vi "Measurement Logic.vi"() -> ()   [LabVIEW 2021, in "adc_fullScaleError.lvlib"]
uses:
  adc_fullScaleError.lvlib
  <instrlib>/niDMM/nidmm.llb/niDMM Function.ctl
  <instrlib>/niDMM/nidmm.llb/niDMM Configure Measurement Digits.vi
  Controls/Sweep Transition Settings.ctl
  <vilib>/DAQmx/configure/timing.llb/DAQmx Timing (Sample Clock).vi
  <vilib>/DAQmx/create/channels.llb/DAQmx Create Channel (AO-Voltage-Basic).vi
  shared/digitalInterface/client/dcvmDPI_AD7606B_client/dcvmDPI_AD7606B_client.lvlib
  <vilib>/gRPC/LabVIEW gRPC Library/Shared/grpcId.ctl
  <vilib>/gRPC/LabVIEW gRPC Library/grpc-lvsupport-release.lvlib
  shared/digitalInterface/client/dcvmDPI_AD7606B_clientImpl/dcvmDPI_AD7606B_clientImpl.lvlib
  Measurement Configuration.ctl
  Measurement Results.ctl
  <vilib>/MeasurementLink/MeasurementLink Measurement Server/Measure Call Context/Measure Call Context.lvclass
panel:
  out "error out":errorcluster
  in  "error in":errorcluster
  out "measurement results":T1
  in  "measurement configuration":T2={"Input channel"=1, "Full scale range"=10.0, "Transition span"=1.5, "Transition step size"=0.05, "Analog source resource name"="", "Digital capture resource name"="", "Digital capture sample rate"=0.0, "Digital capture samples"=10000, "DMM resource name"="", "DMM range"=10.0, "DMM resolution"=5.5} {"DMM range" format="%#_6pV"; "Digital capture sample rate" format="%#_6pS/s"; "Transition step size" format="%#_gLSB"; "Transition span" format="%#_gLSB"; "Full scale range" format="%#_6pV"}
  out "measure call context out":refnum<class "Measure Call Context.lvclass">
  in  "measure call context in":refnum<class "Measure Call Context.lvclass">
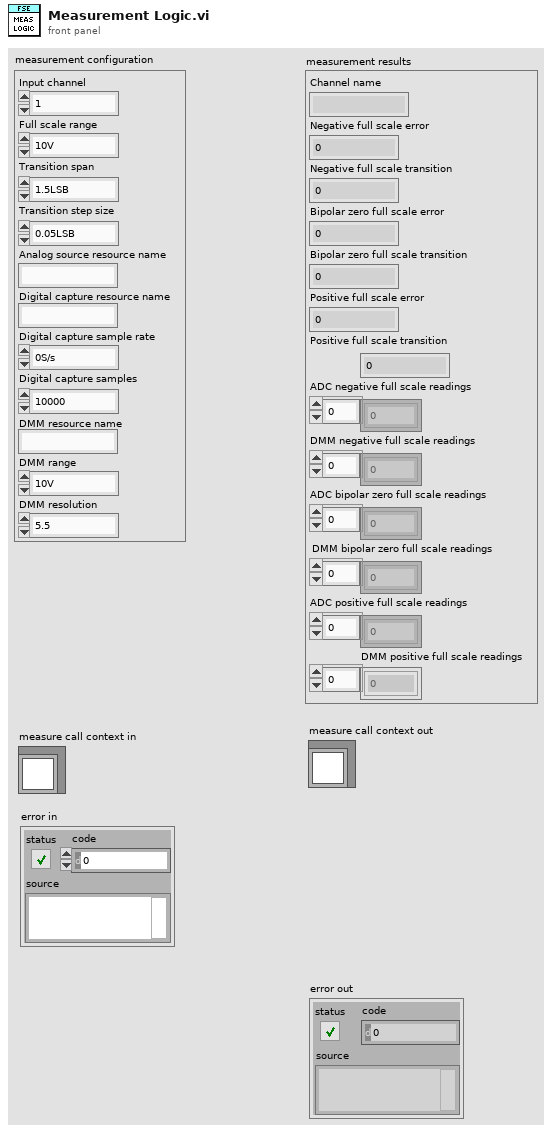
[diagram p1: front panel]
types:
  T1 = typedef "adc_fullScaleError.lvlib/Measurement Results.ctl" = cluster{"Channel name":string, "Negative full scale error":dbl, "Negative full scale transition":dbl, "Bipolar zero full scale error":dbl, "Bipolar zero full scale transition":dbl, "Positive full scale error":dbl, "Positive full scale transition":dbl, "ADC negative full scale readings":dbl[], "DMM negative full scale readings":dbl[], "ADC bipolar zero full scale readings":dbl[], "DMM bipolar zero full scale readings":dbl[], "ADC positive full scale readings":dbl[], "DMM positive full scale readings":dbl[]}
  T2 = typedef "adc_fullScaleError.lvlib/Measurement Configuration.ctl" = cluster{"Input channel":i32, "Full scale range":dbl, "Transition span":dbl, "Transition step size":dbl, "Analog source resource name":string, "Digital capture resource name":string, "Digital capture sample rate":dbl, "Digital capture samples":u32, "DMM resource name":string, "DMM range":dbl, "DMM resolution":dbl}
  T3 = typedef "adc_fullScaleError.lvlib/Sweep Transition Settings.ctl" = cluster{"Gain":dbl, "Offset":dbl, "Slope":dbl, "Intercept":dbl, "Max input":dbl, "Min input":dbl, "Ideal LSB":dbl, "Codes":dbl, "Transition span ":dbl, "Number of steps":i32, "Calibration done":bool}
  T4 = typedef "grpc-lvsupport-release.lvlib/grpcId.ctl" = u64
  T5 = cluster{"DSG Session":refnum<k21>, "DMM Session":refnum<k15>, "gRPC session":T4}
  T6 = typedef "niDMM Function.ctl" = enum16{"DC Volts", "AC Volts", "DC Current", "AC Current", "2-wire Resistance", "4-wire Resistance", "Diode", "Frequency", "Period", "AC Volts DC Coupled", "Capacitance", "Inductance", "Temperature"}
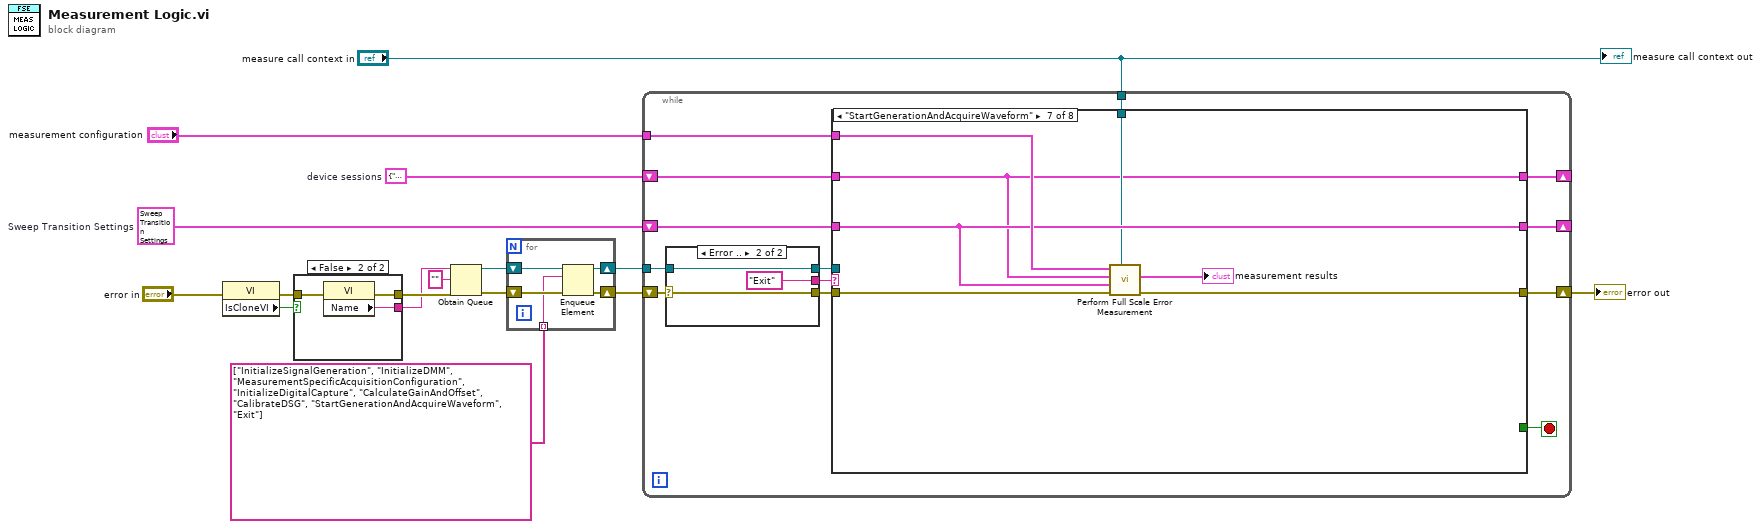
[diagram p0: block diagram]
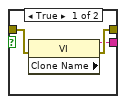
[diagram p2: hidden frame]
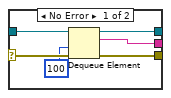
[diagram p3: hidden frame]
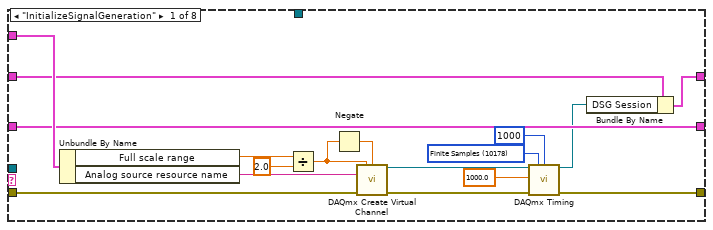
[diagram p4: hidden frame]
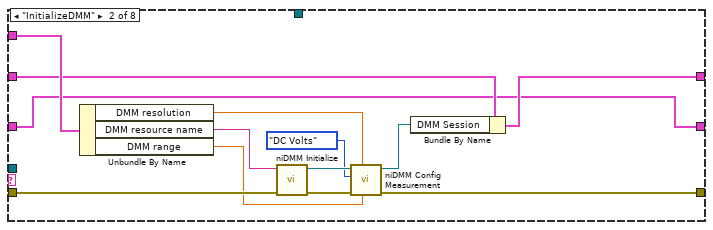
[diagram p5: hidden frame]
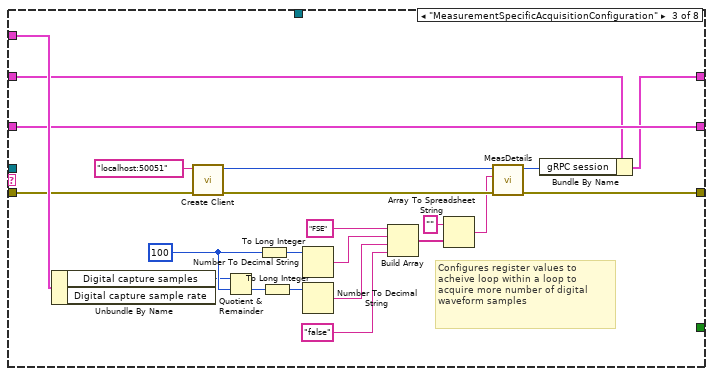
[diagram p6: hidden frame]
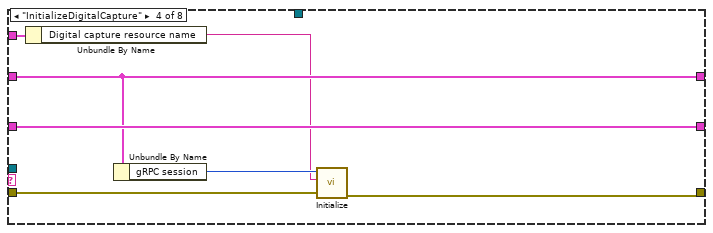
[diagram p7: hidden frame]
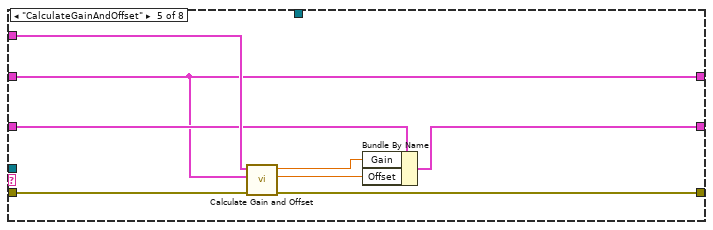
[diagram p8: hidden frame]
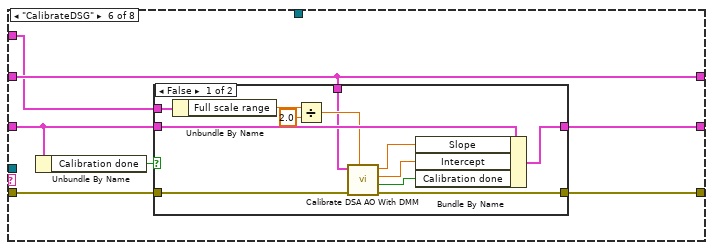
[diagram p9: hidden frame]
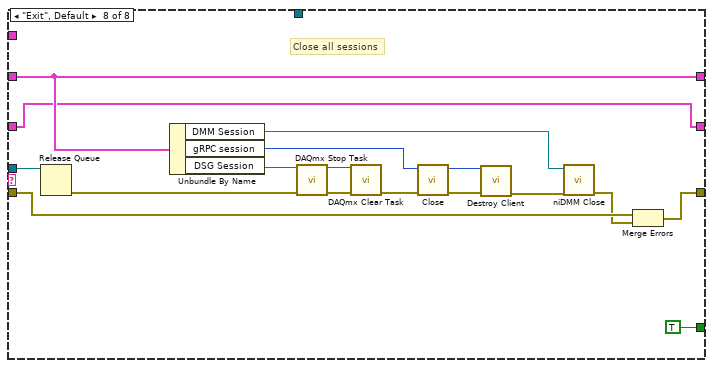
[diagram p11: hidden frame]
diagram:
  w2 = T3 {"Gain"=0.0, "Offset"=0.0, "Slope"=0.0, "Intercept"=0.0, "Max input"=0.0, "Min input"=0.0, "Ideal LSB"=0.0, "Codes"=0.0, "Transition span "=0.0, "Number of steps"=0, "Calibration done"=FALSE}  # Sweep Transition Settings
  w13 = T5 {"DSG Session"="", "DMM Session"="", "gRPC session"=0}  # device sessions
  n1 = property class="VI"(error in="error in") -> (error out=w9:errorcluster, "IsCloneVI"=w10:bool)  [unwired: 1 in, 1 out]
  n2 = case shown="False" w10 {
    tunnel: [w19 w22] -> w7
    tunnel: [w18 w21] -> w6
    tunnel: w9 -> [w17 w20]
    frame True {
      n3 = property class="VI"(error in=w17) -> (error out=w19:errorcluster, "Clone Name"=w18:string)  [unwired: 1 in, 1 out]
    }
    frame False {
      n4 = property class="VI"(error in=w20) -> (error out=w22:errorcluster, "Name"=w21:string)  [unwired: 1 in, 1 out]
    }
  }
  n5 = Obtain Queue(name (unnamed)=w6, element data type="", error in (no error)=w7) -> (queue out=w15:refnum<queue>, error out=w5:errorcluster)  [unwired: 2 in, 1 out]
  n6 = for {
    shift-right: [w25] -> w14
    shift-left: w15 -> [w27]
    shift-right: [w24] -> w4
    shift-left: w5 -> [w26]
    tunnel: string[] ["InitializeSignalGeneration", "InitializeDMM", "MeasurementSpecificAcquisitionConfiguration", "InitializeDigitalCapture", "CalculateGainAndOffset", "CalibrateDSG", "StartGenerationAndAcquireWaveform", "Exit"] ("Step sequence") -> [w23] mode=indexing
    n7 = Enqueue Element(queue=w27, element=w23, error in (no error)=w26) -> (queue out=w25:refnum<queue>, error out=w24:errorcluster)  [unwired: 1 in, 1 out]
  }
  n8 = while {
    tunnel: w14 -> [w35]
    shift-right: [w40] -> w11
    shift-left: w4 -> [w36]
    tunnel: "measurement configuration" -> [w39]
    shift-right: [w37] -> _
    shift-left: w13 -> [w38]
    shift-right: [w30] -> _
    shift-left: w2 -> [w31]
    tunnel: "measure call context in" -> [w28]
    stop <- w29 stop-if-true
    n9 = case shown="Error .." w36 {
      selector: w36 -> [w44 w48]
      tunnel: w35 -> [w46 w47]
      tunnel: [w45 "Exit" ("t")] -> w34
      tunnel: [w43 w48] -> w33
      tunnel: [w41 w47] -> w32
      frame No Error {
        n10 = Dequeue Element(queue=w46, timeout in ms (-1)=100, error in (no error)=w44) -> (queue out=w41:refnum<queue>, element=w45:string, error out=w43:errorcluster)  [unwired: 1 out]
      }
      frame Error {
      }
    }
    n11 = case shown="\"StartGenerationAndAcquireWaveform\"" w34 {
      tunnel: [w64 w71 w80 w102 w116 w119 w141 w154] -> w40
      tunnel: w33 -> [w65 w77 w88 w106 w115 w120 w144 w155]
      tunnel: w39 -> [w63 w79 w100 w108 w114 w117 w142 _]
      tunnel: w38 -> [w53 w70 w83 w105 w109 w118 w138 w158]
      tunnel: [w52 w68 w81 w105 w109 w118 w138 w158] -> w37
      tunnel: w32 -> [_ _ _ _ _ _ _ w157]
      tunnel: w31 -> [w54 w67 w97 w107 w113 w122 w140 w150]
      tunnel: [w54 w67 w97 w107 w110 w121 w140 w150] -> w30
      tunnel: [_ _ _ _ _ _ _ TRUE] -> w29
      tunnel: w28 -> [_ _ _ _ _ _ w139 _]
      frame "InitializeSignalGeneration" {
        w60 = 10178 items=["Finite Samples"=10178, "Continuous Samples"=10123, "Hardware Timed Single Point"=12522] ("sample mode")
        n12 = Unbundle By Name(w63) -> ("Full scale range"=w58:dbl, "Analog source resource name"=w66:string)
        n13 = Divide(x=w58, y=2.0) -> (x/y=w56:dbl)
        n14 = Negate(x=w56) -> (-x=w55:dbl)
        n15 = call-poly <vilib>:"DAQmx Create Virtual Channel.vi"("maximum value"=w56, "minimum value"=w55, "physical channels"=w66, "error in"=w65) -> ("task out"=w62:refnum<k21>, "error out"=w61:errorcluster)  [unwired: 10 in]
        n16 = call-poly <vilib>:"DAQmx Timing.vi"("task/channels in"=w62, "sample mode"=w60, "samples per channel"=1000, "rate"=1000.0, "error in"=w61) -> ("task out"=w51:refnum<k21>, "error out"=w64:errorcluster)  [unwired: 9 in]
        n17 = Bundle By Name(cluster=w53, "DSG Session"=w51) -> (w52:T5)
      }
      frame "InitializeDMM" {
        n18 = Unbundle By Name(w79) -> ("DMM resolution"=w74:dbl, "DMM resource name"=w78:string, "DMM range"=w73:dbl)
        n19 = call <instrlib>:"niDMM Initialize.vi"("error in (no error)"=w77, "Instrument Descriptor"=w78) -> ("error out"=w76:errorcluster, "instrument handle out"=w75:refnum<k15>)  [unwired: 8 in]
        n20 = call-poly <instrlib>:"niDMM Config Measurement.vi"("Range"=w73, "Resolution in Digits"=w74, "error in (no error)"=w76, "Function"=niDMM_Function."DC Volts", "instrument handle"=w75) -> ("error out"=w71:errorcluster, "instrument handle out"=w69:refnum<k15>)  [unwired: 5 in]
        n21 = Bundle By Name(cluster=w70, "DMM Session"=w69) -> (w68:T5)
      }
      frame "MeasurementSpecificAcquisitionConfiguration" {
        w101 = u32 100 ("value")
        # "Configures register values to acheive loop within a loop to acquire more number of digital waveform samples"
        n22 = Unbundle By Name(w100) -> ("Digital capture samples"=w99:u32)  [unwired: 1 out]
        n23 = call "Create Client.vi"("error in"=w88, "address"="localhost:50051") -> ("error out"=w85:errorcluster, "gRPC ID Out"=w86:T4)  [unwired: 8 in]
        n24 = Quotient & Remainder(x=w99, y=w101) -> (floor(x/y)=w98:u32)  [unwired: 1 out]
        n25 = To Long Integer(number=w101) -> (32bit integer=w96:i32)
        n26 = To Long Integer(number=w98) -> (32bit integer=w95:i32)
        n27 = Number To Decimal String(number=w96) -> (decimal integer string=w93:string)  [unwired: 1 in]
        n28 = Number To Decimal String(number=w95) -> (decimal integer string=w92:string)  [unwired: 1 in]
        n29 = Build Array("FSE", w93, w92, "false") -> (w90:string[])
        n30 = Array To Spreadsheet String(array=w90, 3:"" ("format string")) -> (spreadsheet string=w84:string)  [unwired: 1 in]
        n31 = call "MeasDetails.vi"("error in"=w85, "Active measurement"=w84, "gRPC session in"=w86) -> ("error out"=w80:errorcluster, "gRPC session out"=w82:T4)  [unwired: 7 in]
        n32 = Bundle By Name(cluster=w83, "gRPC session"=w82) -> (w81:T5)
      }
      frame "InitializeDigitalCapture" {
        n33 = Unbundle By Name(w108) -> ("Digital capture resource name"=w103:string)
        n34 = Unbundle By Name(w105) -> ("gRPC session"=w104:T4)
        n35 = call "Initialize.vi"("error in"=w106, "Digital capture resource name"=w103, "gRPC session in"=w104) -> ("error out"=w102:errorcluster)  [unwired: 7 in, 1 out]
      }
      frame "CalculateGainAndOffset" {
        n36 = call "Calculate Gain and Offset.vi"("error in"=w115, "device sessions"=w109, "measurement configuration"=w114) -> ("error out"=w116:errorcluster, "Offset"=w111:dbl, "Gain"=w112:dbl)  [unwired: 6 in]
        n37 = Bundle By Name(cluster=w113, "Gain"=w112, "Offset"=w111) -> (w110:T3)
      }
      frame "CalibrateDSG" {
        n38 = Unbundle By Name(w122) -> ("Calibration done"=w123:bool)
        n39 = case shown="False" w123 {
          tunnel: w118 -> [w124 _]
          tunnel: w122 -> [w135 w137]
          tunnel: [w131 w137] -> w121
          tunnel: w120 -> [w130 w136]
          tunnel: [w129 w136] -> w119
          tunnel: w117 -> [w128 _]
          frame False {
            n40 = Unbundle By Name(w128) -> ("Full scale range"=w127:dbl)
            n41 = Divide(x=w127, y=2.0) -> (x/y=w125:dbl)
            n42 = call "Calibrate DSA AO With DMM.vi"("DAQ output range"=w125, "error in"=w130, "device sessions"=w124) -> ("error out"=w129:errorcluster, "Calibration done"=w133:bool, "intercept"=w132:dbl, "slope"=w134:dbl)  [unwired: 5 in]
            n43 = Bundle By Name(cluster=w135, "Slope"=w134, "Intercept"=w132, "Calibration done"=w133) -> (w131:T3)
          }
          frame True {
          }
        }
      }
      frame "StartGenerationAndAcquireWaveform" {
        n44 = call "Perform Full Scale Error Measurement.vi"("Measurement Context"=w139, "error in"=w144, "Sweep transition settings"=w140, "device sessions"=w138, "measurement configuration"=w142) -> ("error out"=w141:errorcluster, "measurement results out"=→"measurement results":T1)  [unwired: 5 in]
      }
      frame "Exit", Default {
        (unwired) TRUE
        # "Close all sessions"
        n45 = Release Queue(queue=w157) -> (error out=w156:errorcluster)  [unwired: 2 in, 2 out]
        n46 = Unbundle By Name(w158) -> ("DMM Session"=w152:refnum<k15>, "gRPC session"=w148:T4, "DSG Session"=w161:refnum<k21>)
        n47 = call <vilib>:"DAQmx Stop Task.vi"("task/channels in"=w161, "error in"=w156) -> ("task out"=w160:refnum<k21>, "error out"=w159:errorcluster)  [unwired: 12 in]
        n48 = call <vilib>:"DAQmx Clear Task.vi"("task in"=w160, "error in"=w159) -> ("error out"=w149:errorcluster)  [unwired: 13 in]
        n49 = call "Close.vi"("error in"=w149, "gRPC session in"=w148) -> ("error out"=w146:errorcluster, "gRPC session out"=w147:T4)  [unwired: 8 in]
        n50 = call "Destroy Client.vi"("error in"=w146, "gRPC ID"=w147) -> ("error out"=w145:errorcluster)  [unwired: 9 in]
        n51 = call <instrlib>:"niDMM Close.vi"("error in (no error)"=w145, "instrument handle"=w152) -> ("error out"=w153:errorcluster)  [unwired: 9 in]
        n52 = Merge Errors(w155, w153) -> (w154:errorcluster)
      }
    }
  }
  "error out" <- w11
  "measure call context out" <- "measure call context in"
